vi "mxTaskCleared.vi"(1 "task in":refnum<k21>) -> (0 "Task Cleared":bool)   [LabVIEW 2010]
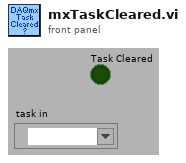
[diagram p1: front panel]
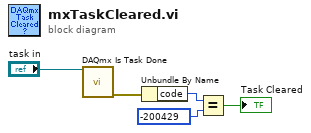
[diagram p0: block diagram]
diagram:
  n1 = call <vilib>:"DAQmx Is Task Done.vi"("task/channels in"="task in") -> ("error out"=w3:errorcluster)  [unwired: 12 in, 2 out]
  n2 = Unbundle By Name(w3) -> ("code"=w5:i32)
  n3 = Equal?(x=w5, y=-200429) -> (x = y?=→"Task Cleared":bool)
